vi "Authentication.vi"(8 "error in (no error)":errorcluster) -> (0 "error out":errorcluster, 3 "Match?":bool)   [LabVIEW 2016, in "User Interface.lvlib"]
uses:
  User Interface.lvlib
  Authentication State.ctl
  Action log.ctl
  Database/Class/DB/Credential.ctl
  Database/Database.lvlib
panel:
  out "Time 2":string="Authentication"
  out "Msg Out":string
  in  "Password":string
  in  "Username":string(combo)
  in  "User Level":string(combo)
  in  "Cancel":bool
  in  "Delete":bool
  in  "Add":bool
  in  "Edit":bool
  in  "Authentication Tab":enum32{"User", "Edit User"}(tab)
  in  "User Name":string(combo)
  in  "Password":string
  in  "Log":bool
  out "Time":string="Sat  8/3/2019  8:10:44 PM"
  in  "Update":bool
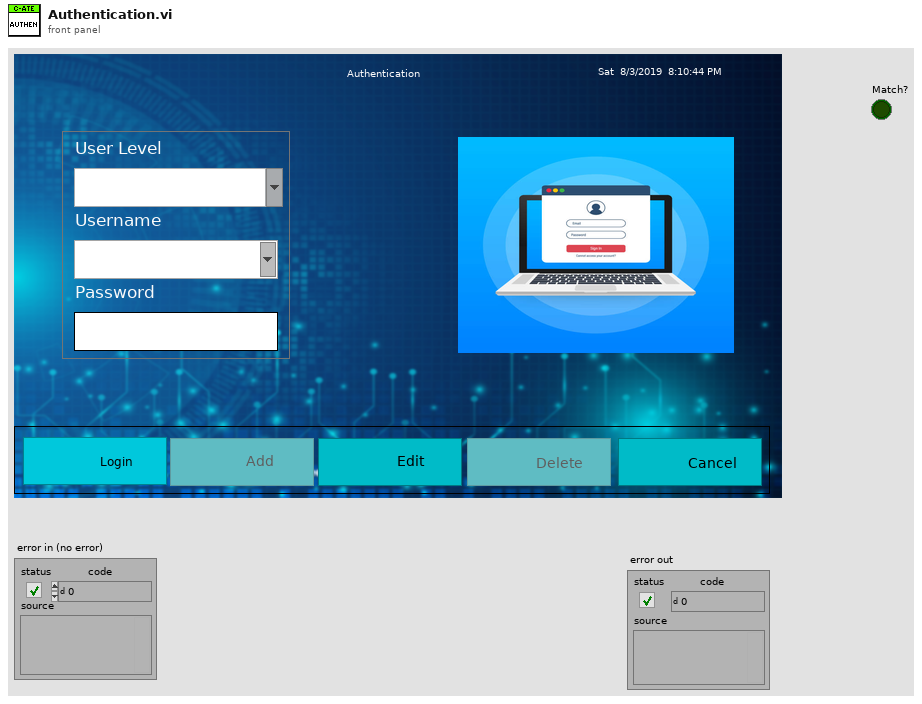
[diagram p1: front panel]
types:
  T1 = typedef "User Interface.lvlib/Authentication State.ctl" = enum16{"Initialize", "Main", "Add User", "Delete User", "Close"}
  T2 = typedef "User Interface.lvlib/Action log.ctl" = enum16{"Init", "Read", "Write", "Close"}
  T3 = typedef "Database.lvlib/Credential.ctl" = cluster{"User Level":string, "User Name":string, "Password":string}
  T4 = enum8{"Enabled", "Disabled", "Disabled and Grayed Out"}
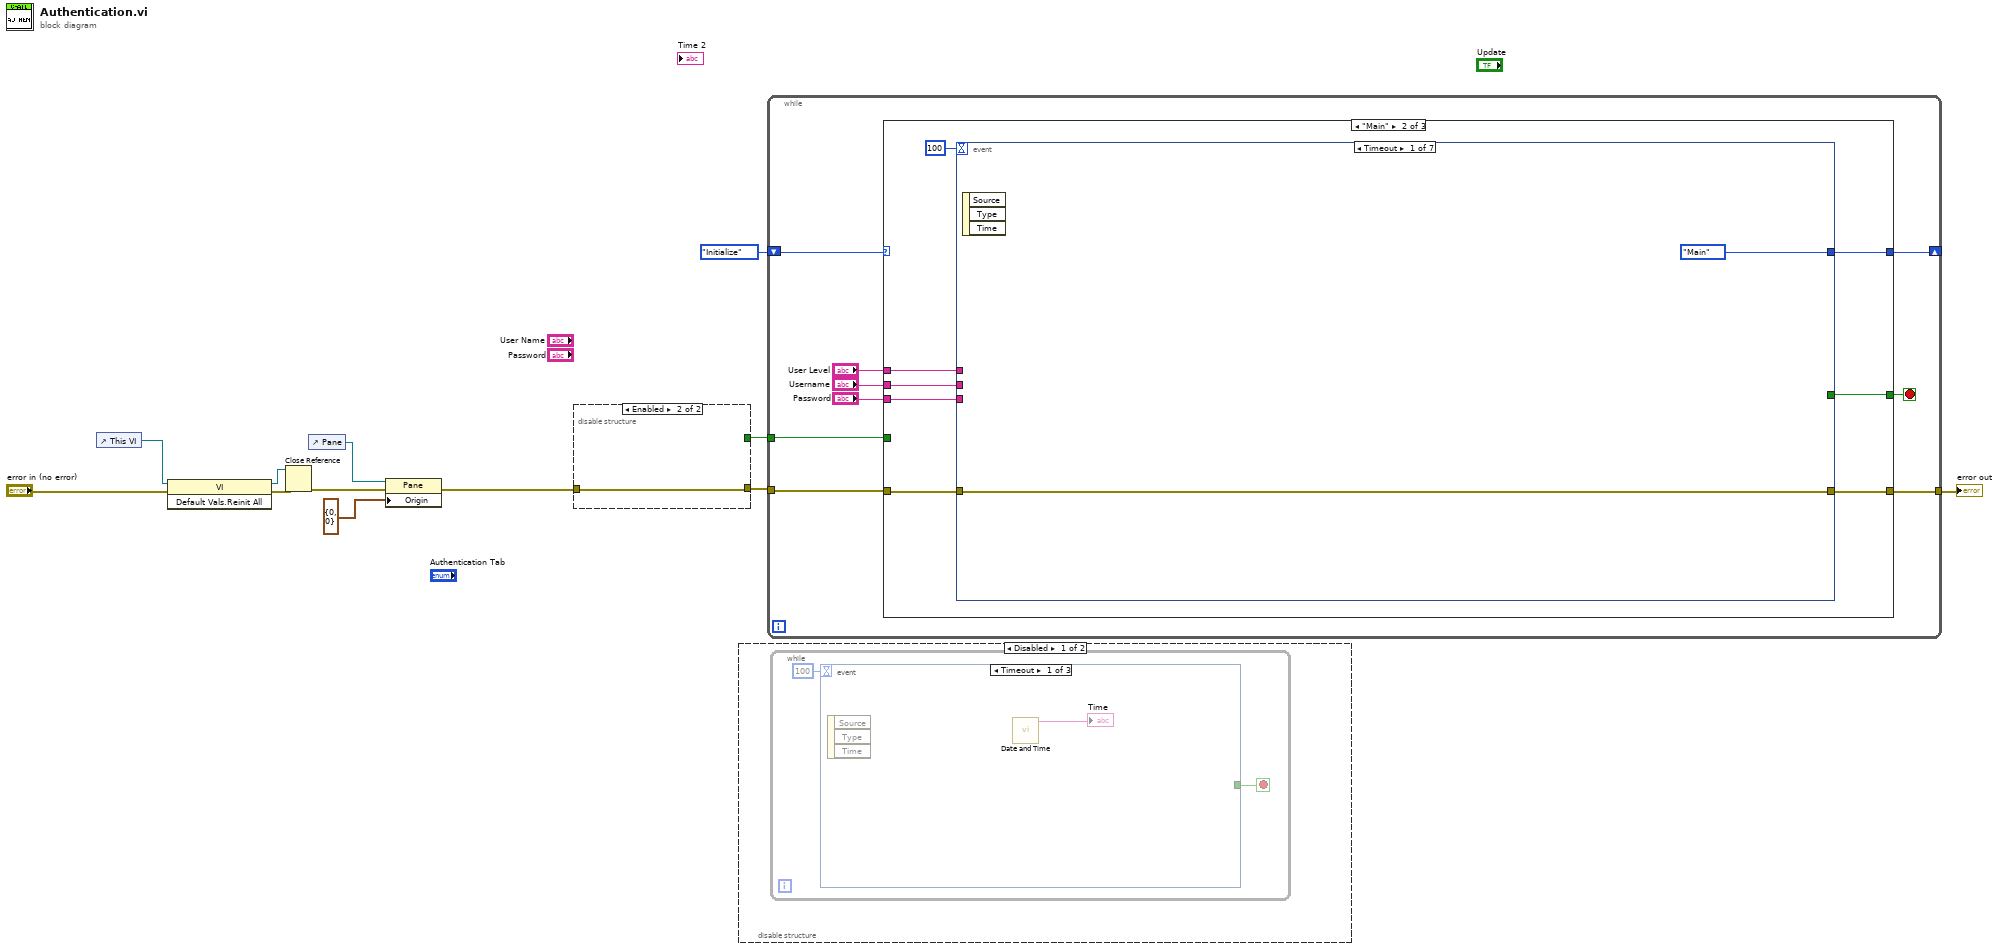
[diagram p0: block diagram]
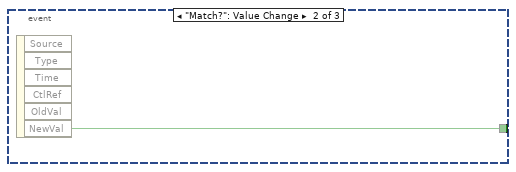
[diagram p2: hidden frame]
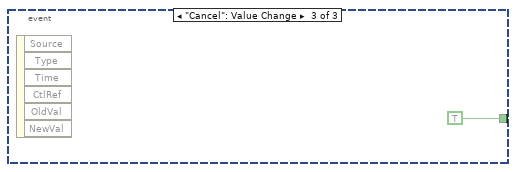
[diagram p3: hidden frame]
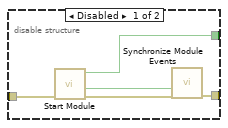
[diagram p5: hidden frame]
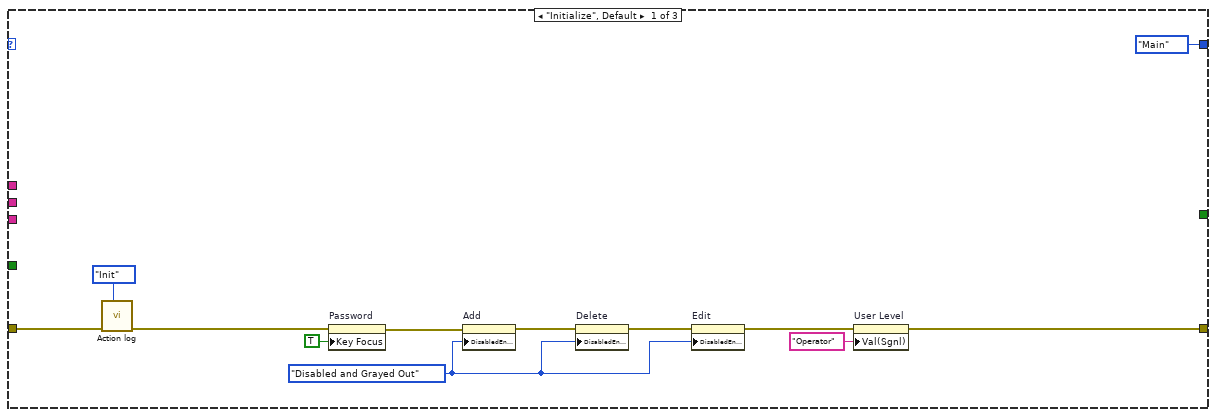
[diagram p6: hidden frame]
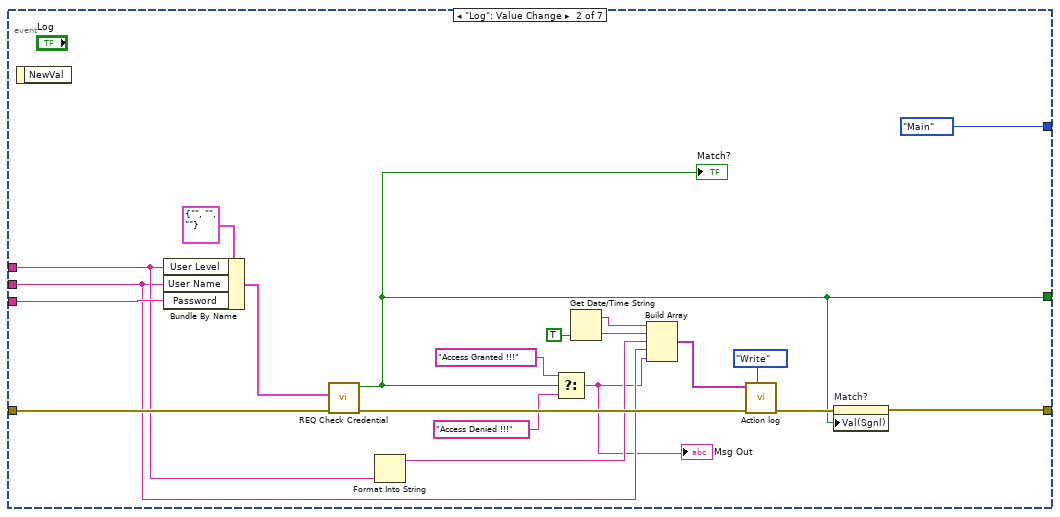
[diagram p7: hidden frame]
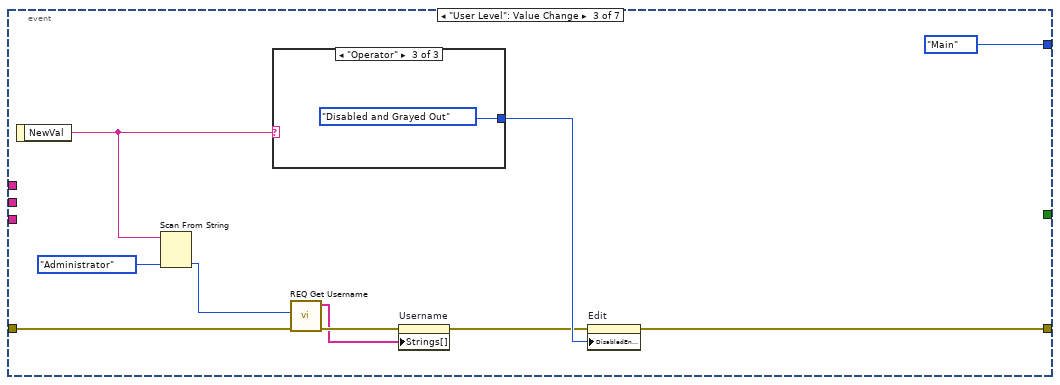
[diagram p8: hidden frame]
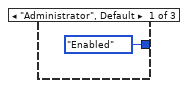
[diagram p9: hidden frame]
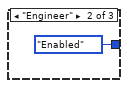
[diagram p10: hidden frame]
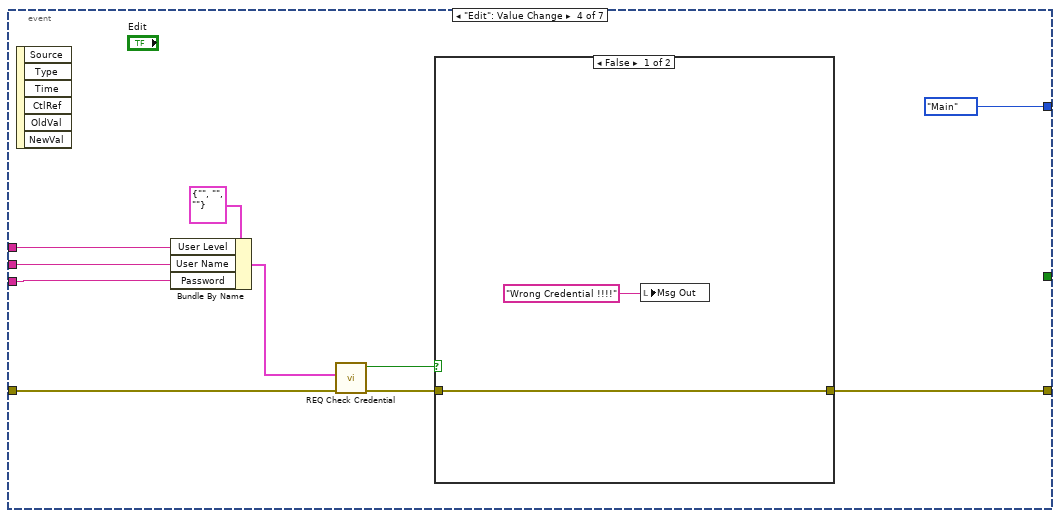
[diagram p11: hidden frame]
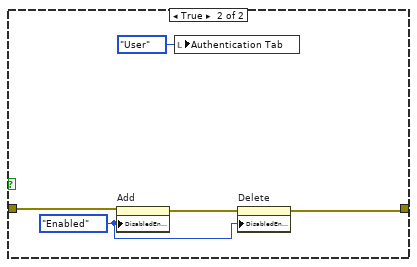
[diagram p12: hidden frame]
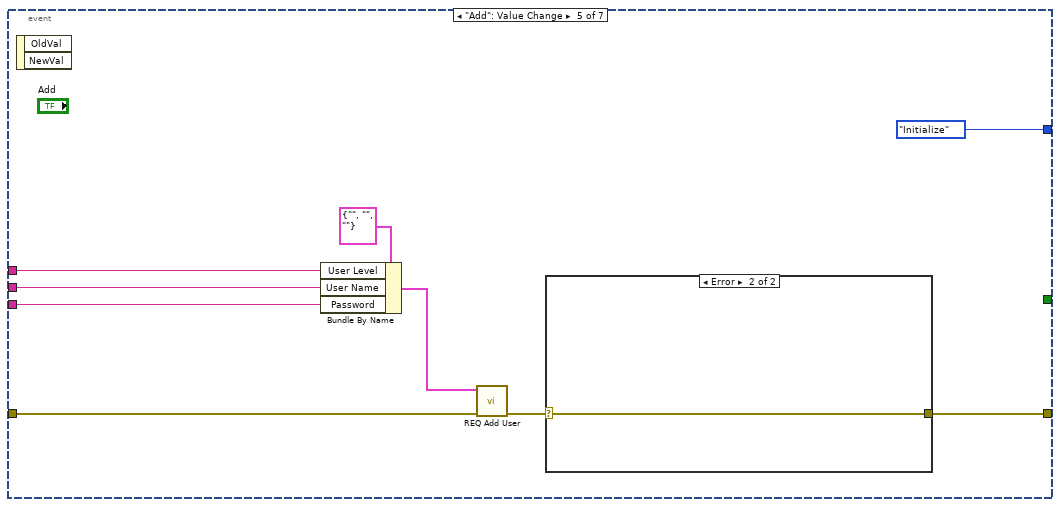
[diagram p13: hidden frame]
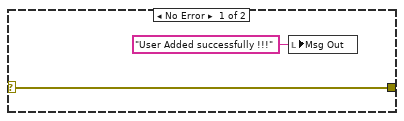
[diagram p14: hidden frame]
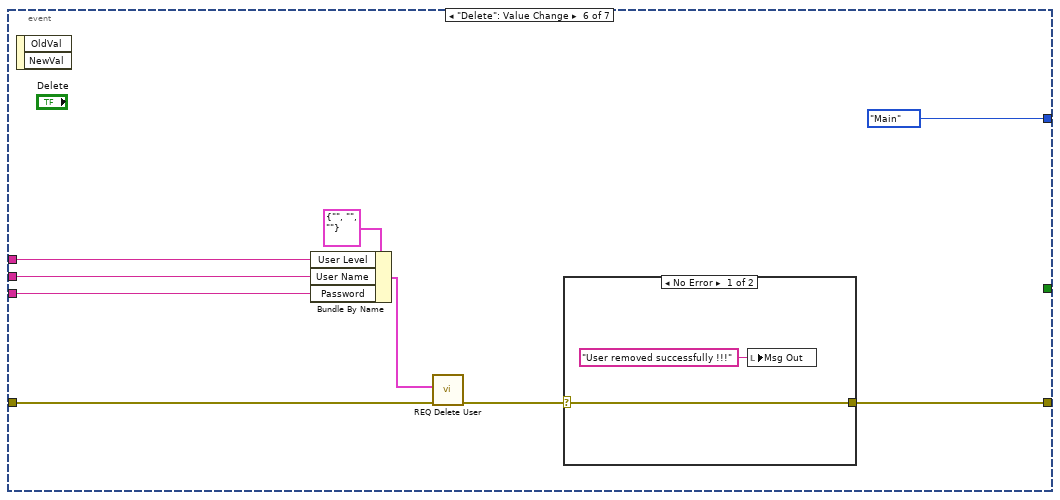
[diagram p15: hidden frame]
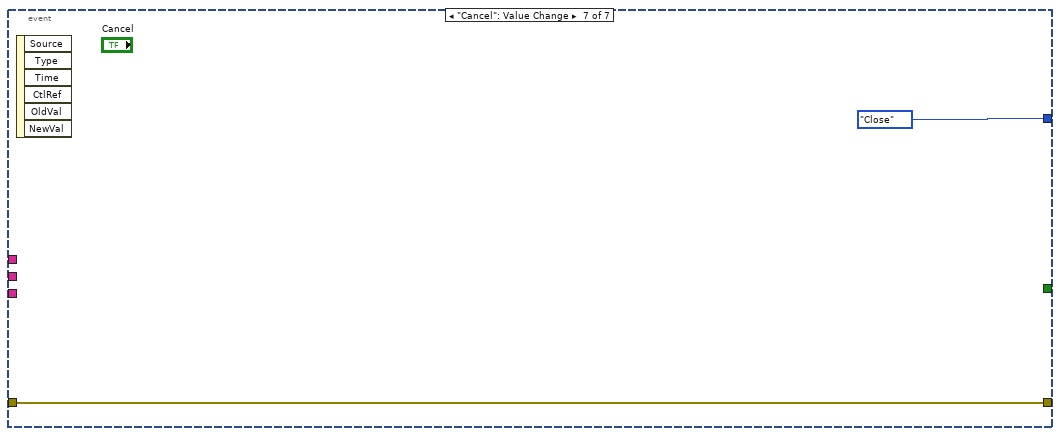
[diagram p17: hidden frame]
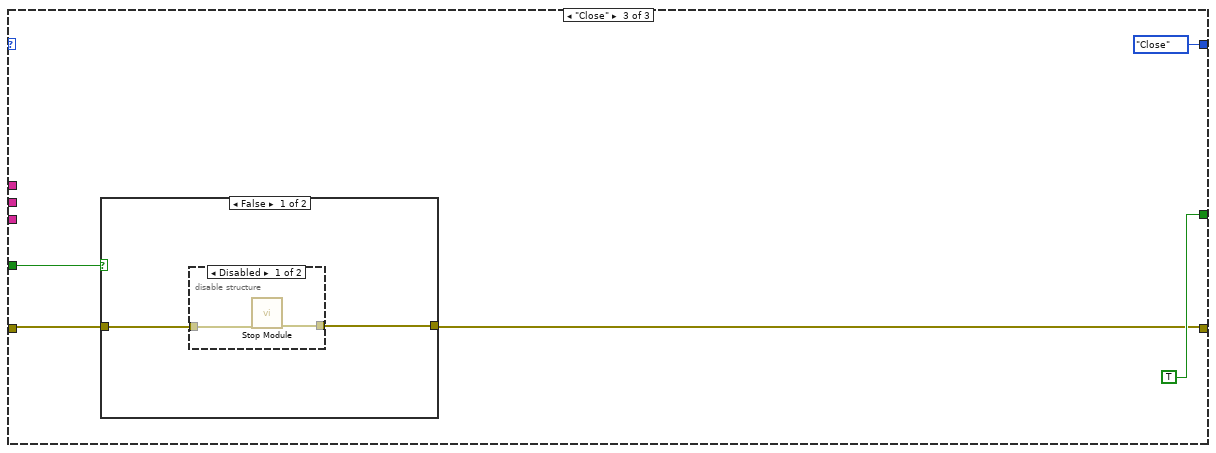
[diagram p18: hidden frame]
diagram:
  n1 = control-ref of="This VI"() -> (w10:refnum<vi>)
  n2 = invoke class="VI" method="Default Vals.Reinit All"(reference=w10, error in="error in (no error)") -> (reference out=w8:refnum<vi>, error out=w9:errorcluster)  [unwired: 1 in, 1 out]
  n3 = Close Reference(reference=w8, error in (no error)=w9) -> (error out=w7:errorcluster)
  n4 = control-ref of="Pane"() -> (w4:refnum<vi>)
  n5 = property class="Pane"(reference=w4, error in=w7, "Origin"=cluster{"Horizontal":i16, "Verticle":i16} {"Horizontal"=0, "Verticle"=0} ("Origin (0,0)")) -> (error out=w3:errorcluster)  [unwired: 1 out]
  n6 = disable-structure shown="Enabled" {
    disable-tunnel: w3 -> [w15 w18]
    disable-tunnel: [w14 w18] -> w2
    disable-tunnel: [w13 _] -> w1
    frame Disabled {
      n7 = call "Start Module.vi"("error in"=w15) -> ("error out"=w16:errorcluster, "Wait for Event Sync?"=w17:bool, "Module Was Already Running?"=w13:bool)  [unwired: 7 in, 1 out]
      n8 = call "Synchronize Module Events.vi"("error in"=w16, "Wait for Event Sync?"=w17) -> ("error out"=w14:errorcluster)  [unwired: 9 in]
    }
    frame Enabled {
    }
  }
  n9 = disable-structure shown="Disabled" {
    frame Disabled {
      n10 = while {
        stop <- w19 stop-if-true
        n11 = event shown="[0] Timeout" {
          selector: _ -> [_ _ _]
          dyn-events: _ -> [_ _ _]
          timeout: 100 -> [_ _ _]
          tunnel: [_ w22 TRUE] -> w19
          event Timeout {
            n12 = event-data() -> ()  [unwired: 1 in, 3 out]
            n13 = call "Date and Time.vi"() -> ("Current Time"=→"Time":string)  [unwired: 11 in]
          }
          event "Match?": Value Change {
            n14 = event-data() -> ("NewVal"=w22:bool)  [unwired: 1 in, 5 out]
          }
          event "Cancel": Value Change {
            n15 = event-data() -> ()  [unwired: 1 in, 6 out]
          }
        }
      }
    }
    frame Enabled {
    }
  }
  n16 = while {
    shift-right: [w29] -> _
    shift-left: Authentication_State."Initialize" -> [w32]
    tunnel: w2 -> [w31]
    tunnel: [w30] -> w11
    tunnel: w1 -> [w27]
    stop <- w28 stop-if-true
    n17 = case shown="\"Main\"" w32 {
      tunnel: w31 -> [w38 w52 w132]
      tunnel: [w34 w50 w131] -> w30
      tunnel: [Authentication_State."Main" w51 Authentication_State."Close"] -> w29
      tunnel: [_ w45 TRUE] -> w28
      tunnel: "User Level" -> [_ w48 _]
      tunnel: "Username" -> [_ w47 _]
      tunnel: "Password" -> [_ w46 _]
      tunnel: w27 -> [_ _ w133]
      frame "Initialize", Default {
        w41 = T4."Disabled and Grayed Out" ("Disabled")
        n18 = call "Action log.vi"("Command"=Action_log."Init", "error in (no error)"=w38) -> ("error out"=w36:errorcluster)  [unwired: 9 in]
        n19 = property on="Password" class="Str"(error in=w36, "Key Focus"=TRUE) -> (error out=w39:errorcluster)  [unwired: 1 in, 1 out]
        n20 = property on="Add" class="Bool"(error in=w39, "DisabledEnum"=w41) -> (error out=w43:errorcluster)  [unwired: 1 in, 1 out]
        n21 = property on="Delete" class="Bool"(error in=w43, "DisabledEnum"=w41) -> (error out=w42:errorcluster)  [unwired: 1 in, 1 out]
        n22 = property on="Edit" class="Bool"(error in=w42, "DisabledEnum"=w41) -> (error out=w35:errorcluster)  [unwired: 1 in, 1 out]
        n23 = property on="User Level" class="CmbBox"(error in=w35, "Val(Sgnl)"="Operator" ("Value (Signaling)")) -> (error out=w34:errorcluster)  [unwired: 1 in, 1 out]
      }
      frame "Main" {
        n24 = event shown="[0] Timeout" {
          selector: _ -> [_ _ _ _ _ _ _]
          dyn-events: _ -> [_ _ _ _ _ _ _]
          timeout: 100 -> [_ _ _ _ _ _ _]
          tunnel: w52 -> [w53 w74 w82 w94 w112 w122 w129]
          tunnel: [Authentication_State."Main" Authentication_State."Main" Authentication_State."Main" Authentication_State."Main" Authentication_State."Initialize" Authentication_State."Main" Authentication_State."Close"] -> w51
          tunnel: [w53 w56 w81 w88 w105 w117 w129] -> w50
          tunnel: w48 -> [_ w64 _ w93 w109 w121 _]
          tunnel: w47 -> [_ w59 _ w92 w108 w120 _]
          tunnel: w46 -> [_ w72 _ w91 w107 w119 _]
          tunnel: [_ w55 _ _ _ _ _] -> w45
          event Timeout {
            n25 = event-data() -> ()  [unwired: 1 in, 3 out]
          }
          event "Log": Value Change {
            n26 = event-data() -> ()  [unwired: 1 in, 1 out]
            n27 = Bundle By Name(cluster=T3 {"User Level"="", "User Name"="", "Password"=""} ("Credential"), "User Level"=w64, "User Name"=w59, "Password"=w72) -> (w70:T3)
            n28 = call "REQ Check Credential.vi"("error in"=w74, "Credential"=w70) -> ("error out"=w68:errorcluster, "Match?"=w55:bool)  [unwired: 7 in, 1 out]
            "Match?" <- w55
            n29 = Format Into String(w64) -> (resulting string=w60:string)  [unwired: 3 in, 1 out]
            n30 = Select(t="Access Granted !!!", s=w55, f="Access Denied !!!") -> (s? t:f=w58:string)
            "Msg Out" <- w58
            n31 = Get Date/Time String(want seconds? (F)=TRUE) -> (date string=w66:string, time string=w65:string)  [unwired: 2 in]
            n32 = Build Array(w66, w65, w60, w59, w58) -> (w61:string[])
            n33 = call "Action log.vi"("Command"=Action_log."Write", "error in (no error)"=w68, "Data"=w61) -> ("error out"=w57:errorcluster)  [unwired: 8 in]
            n34 = property on="Match?" class="Bool (strict)"(error in=w57, "Val(Sgnl)"=w55) -> (error out=w56:errorcluster)  [unwired: 1 in, 1 out]
          }
          event "User Level": Value Change {
            n35 = event-data() -> ("NewVal"=w79:string)  [unwired: 1 in]
            n36 = Scan From String(input string=w79, default 1=enum16{"Administrator", "Engineer", "Operator"}."Administrator" ("User Level")) -> (output 1=w78:enum16{"Administrator", "Engineer", "Operator"})  [unwired: 3 in, 3 out]
            n37 = case shown="\"Operator\"" w79 {
              tunnel: [T4."Enabled" ("Disabled") T4."Enabled" ("Disabled") T4."Disabled and Grayed Out" ("Disabled")] -> w83
              frame "Administrator", Default {
              }
              frame "Engineer" {
              }
              frame "Operator" {
              }
            }
            n38 = call "REQ Get Username.vi"("error in"=w82, "User Level"=w78) -> ("error out"=w77:errorcluster, "Username"=w75:string[])  [unwired: 7 in, 1 out]
            n39 = property on="Username" class="CmbBox"(error in=w77, "Strings[]"=w75) -> (error out=w76:errorcluster)  [unwired: 1 in, 1 out]
            n40 = property on="Edit" class="Bool"(error in=w76, "DisabledEnum"=w83) -> (error out=w81:errorcluster)  [unwired: 1 in, 1 out]
          }
          event "Edit": Value Change {
            n41 = event-data() -> ()  [unwired: 1 in, 6 out]
            n42 = Bundle By Name(cluster=T3 {"User Level"="", "User Name"="", "Password"=""} ("Credential"), "User Level"=w93, "User Name"=w92, "Password"=w91) -> (w95:T3)
            n43 = call "REQ Check Credential.vi"("error in"=w94, "Credential"=w95) -> ("error out"=w89:errorcluster, "Match?"=w90:bool)  [unwired: 7 in, 1 out]
            n44 = case shown="False" w90 {
              tunnel: w89 -> [w99 w101]
              tunnel: [w99 w100] -> w88
              frame False {
                n45 = local write "Msg Out"("Wrong Credential !!!!" ("message")) -> ()
              }
              frame True {
                w102 = T4."Enabled" ("Disabled")
                n46 = property on="Add" class="Bool"(error in=w101, "DisabledEnum"=w102) -> (error out=w103:errorcluster)  [unwired: 1 in, 1 out]
                n47 = local write "Authentication Tab"(enum32{"User", "Edit User"}."User" ("Authentication Tab")) -> ()
                n48 = property on="Delete" class="Bool"(error in=w103, "DisabledEnum"=w102) -> (error out=w100:errorcluster)  [unwired: 1 in, 1 out]
              }
            }
          }
          event "Add": Value Change {
            n49 = event-data() -> ()  [unwired: 1 in, 2 out]
            n50 = Bundle By Name(cluster=T3 {"User Level"="", "User Name"="", "Password"=""} ("Credential"), "User Level"=w109, "User Name"=w108, "Password"=w107) -> (w110:T3)
            n51 = call "REQ Add User.vi"("error in"=w112, "Credential"=w110) -> ("error out"=w106:errorcluster)  [unwired: 9 in]
            n52 = case shown="Error" w106 {
              selector: w106 -> [w114 w116]
              tunnel: [w114 w116] -> w105
              frame No Error {
                n53 = local write "Msg Out"("User Added successfully !!!" ("Msg Out")) -> ()
              }
              frame Error {
              }
            }
          }
          event "Delete": Value Change {
            n54 = event-data() -> ()  [unwired: 1 in, 2 out]
            n55 = Bundle By Name(cluster=T3 {"User Level"="", "User Name"="", "Password"=""} ("Credential"), "User Level"=w121, "User Name"=w120, "Password"=w119) -> (w123:T3)
            n56 = call "REQ Delete User.vi"("error in"=w122, "Credential"=w123) -> ("error out"=w118:errorcluster)  [unwired: 9 in]
            n57 = case shown="No Error" w118 {
              selector: w118 -> [w126 w128]
              tunnel: [w126 w128] -> w117
              frame No Error {
                n58 = local write "Msg Out"("User removed successfully !!!" ("Msg Out")) -> ()
              }
              frame Error {
              }
            }
          }
          event "Cancel": Value Change {
            n59 = event-data() -> ()  [unwired: 1 in, 6 out]
          }
        }
      }
      frame "Close" {
        n60 = case shown="False" w133 {
          tunnel: w132 -> [w137 w140]
          tunnel: [w136 w140] -> w131
          frame False {
            n61 = disable-structure shown="Disabled" {
              disable-tunnel: w137 -> [w139 _]
              disable-tunnel: [w138 _] -> w136
              frame Disabled {
                n62 = call "Stop Module.vi"("error in"=w139) -> ("error out"=w138:errorcluster)  [unwired: 10 in]
              }
              frame Enabled {
              }
            }
          }
          frame True {
          }
        }
      }
    }
  }
  "error out" <- w11
